vi "Datasocket（上课 从）.vi"() -> ()   [LabVIEW 2017]
panel:
  out "波形图":dbl[](graph)
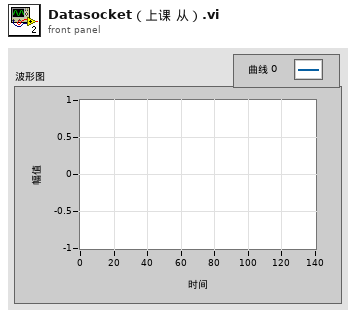
[diagram p1: front panel]
types:
  T1 = cluster{"等待时间（毫秒）":u32, "Sinusoidal Pattern":dbl[], "停止":bool}
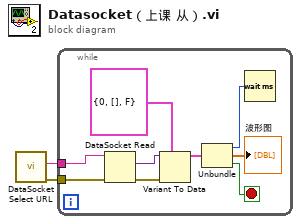
[diagram p0: block diagram]
diagram:
  n1 = call <vilib>:"DataSocket Select URL.vi"() -> ("error out"=w1:errorcluster, "URL"=w2:string)  [unwired: 9 in, 1 out]
  n2 = while {
    tunnel: w2 -> [w5]
    tunnel: w1 -> [w4]
    stop <- w7 stop-if-true
    n3 = DataSocket Read(8:w4, 11:w5) -> (0:w3:errorcluster, 2:w10:variant)  [unwired: 3 in, 5 out]
    n4 = Variant To Data(error in=w3, type=T1 {"等待时间（毫秒）"=0, "Sinusoidal Pattern"=[], "停止"=FALSE} ("输出簇"), Variant=w10) -> (data=w9:T1)  [unwired: 1 out]
    n5 = Unbundle(w9) -> ("等待时间（毫秒）"=w8:u32, "Sinusoidal Pattern"=→"波形图":dbl[], "停止"=w7:bool)
    n6 = Wait (ms)(milliseconds to wait=w8) -> ()  [unwired: 1 out]
  }
